vi "Begin.vi"(8 "error in":errorcluster) -> (0 "error out":errorcluster)   [LabVIEW 2014]
doc: "Called before other user functions, this VI is expected to open initial I/O refnums, load in file data, and do all program initialization. Notice that the <B>error out</B> terminal is simply used for data flow. Wiring it to other structures or subVIs ensures that this VI runs first."
uses:
  <vilib>/Rock Robotics/SystemInterfaces/AI/FPGA_AIChannel.ctl
  <vilib>/Rock Robotics/WPI/Solenoid/WPI_SolenoidChannel.ctl
  navX-MXP Library/SERIAL/IO/NI WPI/WPI_SerialPort_USB.ctl
  <vilib>/Rock Robotics/WPI/SafetyOutput/WPI_SafetyOutputConfigMenu.ctl
  <vilib>/Rock Robotics/WPI/Joystick/WPI_JoystickDeviceEnum.ctl
  <vilib>/Rock Robotics/WPI/Compressor/WPI_CompressorGetSetRefNum.vi
  <vilib>/Rock Robotics/WPI/RobotDrive/WPI_RobotDriveOpen4MotorWithCANTalonSRX.vi
  <vilib>/Rock Robotics/WPI/MotorControl/WPI_MotorControlOpenCANTalonSRX.vi
  <vilib>/Rock Robotics/WPI/Solenoid/WPI_SolenoidOpenSingle.vi
  Robot Global Data.vi
  navX-MXP Library/navX-MXP IMU.lvlib
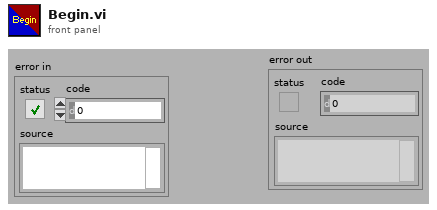
[diagram p1: front panel]
types:
  T1 = typedef "WPI_SolenoidChannel.ctl" = enum8{"Solenoid 0", "Solenoid 1", "Solenoid 2", "Solenoid 3", "Solenoid 4", "Solenoid 5", "Solenoid 6", "Solenoid 7", "Invalid"}
  T2 = typedef "WPI_SolenoidDevRef.ctl" = cluster{"DevStatus":errorcluster, "Pneumatics Control Module":u8, "Forward Solenoid Channel":T1, "Reverse Solenoid Channel":T1}
  T3 = cluster{"String Potentiometer":dbl, "Setpoint":dbl, "Level":sgl}
  T4 = typedef "WPI_CompressorDevRef.ctl" = cluster{"DevStatus":errorcluster, "Pneumatics Control Module":u8}
  T5 = typedef "navX-MXP IMU.lvlib/WPI_SerialPort_USB.ctl" = enum16{"Onboard RS-232", "MXP TTL", "USB"}
  T6 = typedef "navX-MXP IMU.lvlib/navX SPI DevRef.ctl" = cluster{"SPIDevRef":T7, "Board Information":T10, "Status":T11, "Offsets":cluster{"Yaw":dbl, "Quat W":dbl, "Quat X":dbl, "Quat Y":dbl, "Quat Z":dbl}, "Update Rate (4Hz-60Hz)":u8, "refnum name":string, "error":errorcluster}
  T7 = typedef "WPI_SPIDevRef.ctl" = cluster{"DevStatus":errorcluster, "Handle":i32, "Controller":T8, "SPI Bus":T9}
  T8 = typedef "FPGA_TypedefDigitalModule.ctl" = enum16{"Controller 1"}
  T9 = typedef "spi_bus.ctl" = enum16{"SPI On-Board, CS0", "SPI On-Board, CS1", "SPI On-Board, CS2", "SPI On-Board, CS3", "SPI MXP", "Invalid"}
  T10 = typedef "navX-MXP IMU.lvlib/navX Board Information.ctl" = cluster{"WhoAmI (50 | 0x32)":u8, "Board Revision":u8, "Firmware Major Version":u8, "Firmware Minor Version":u8}
  T11 = typedef "navX-MXP IMU.lvlib/navX Status Data.ctl" = cluster{"Update Rate Hz":u8, "Accelerometer Full-Scale Range":u8, "Gyro Full-Scale Range":u16, "NAVX_OP_STATUS":T12, "NAVX_CAL_STATUS":T13, "NAVX_SELFTEST_STATUS":u8, "NAVX_SENSOR_STATUS":T14}
  T12 = typedef "navX-MXP IMU.lvlib/navX NAVX_OP_STATUS.ctl" = u8
  T13 = typedef "navX-MXP IMU.lvlib/navX NAVX_CAL_STATUS.ctl" = u8
  T14 = typedef "navX-MXP IMU.lvlib/navX NAVX_SENSOR_STATUS.ctl" = cluster{"MOVING":bool, "YAW_STABLE":bool, "MAG_DISTURBANCE":bool, "ALTITUDE_VALID":bool, "SEALEVEL_PRESS_SET":bool, "FUSED_HEADING_VALID":bool}
  T15 = typedef "navX-MXP IMU.lvlib/navX Serial DevRef.ctl" = cluster{"SerialPortRef":T16, "Board Information":T10, "Status":T11, "Offsets":cluster{"Yaw":dbl, "Quat W":dbl, "Quat X":dbl, "Quat Y":dbl, "Quat Z":dbl}, "Update Rate (4Hz-60Hz)":u8, "Nav6Mode (YPR)":T17, "refnum name":string, "error":errorcluster}
  T16 = typedef "WPI_SerialPortRef.ctl" = cluster{"DevStatus":errorcluster, "Serial Port Name":refnum<visa-resource-name>}
  T17 = typedef "navX-MXP IMU.lvlib/navX Serial Mode.ctl" = enum16{"YPR", "Gyro", "Quaternion"}
  T18 = typedef "FPGA_AIChannel.ctl" = enum8{"AI 0", "AI 1", "AI 2", "AI 3", "AI MXP 0", "AI MXP 1", "AI MXP 2", "AI MXP 3", "Invalid"}
  T19 = typedef "WPI_AnalogChannelDevRef.ctl" = cluster{"DevStatus":errorcluster, "Controller":T20, "Analog Channel":T18}
  T20 = typedef "FPGA_TypedefAnalogModule.ctl" = enum16{"Controller 1"}
  T21 = typedef "WPI_SafetyOutputConfigMenu.ctl" = enum16{"Enable", "Disable"}
  T22 = typedef "WPI_RobotDriveDevRef.ctl" = cluster{"DevStatus":errorcluster, "Motors[]":T23[], "Square Inputs":bool, "Max Output":dbl}
  T23 = typedef "WPI_MotorControlDeviceRef.ctl" = cluster{"DeviceStatus":errorcluster, "Type":T24, "PWM":cluster{"Controller":T8, "PWM Channel":T25, "DeadBand":T26}, "CAN":cluster{"Device Number":u8, "Control Mode":T27, "Semaphore":T28, "Max Vout":dbl, "TalonSRX Control Mode":T29}, "Invert":bool, "TransformRef":T30, "InvTransformRef":T30}
  T24 = typedef "WPI_MotorControlType.ctl" = enum16{"PWM", "CAN", "CANTalonSRX"}
  T25 = typedef "FPGA_DIOPWMChannel.ctl" = enum8{"PWM 0", "PWM 1", "PWM 2", "PWM 3", "PWM 4", "PWM 5", "PWM 6", "PWM 7", "PWM 8", "PWM 9", "PWM MXP 0", "PWM MXP 1", "PWM MXP 2", "PWM MXP 3", "PWM MXP 4", "PWM MXP 5", "PWM MXP 6", "PWM MXP 7", "PWM MXP 8", "PWM MXP 9", "Invalid"}
  T26 = typedef "WPI_PWMDeadband.ctl" = cluster{"Name":string, "maxPositivePwm":i32, "minPositivePwm":i32, "centerPwm":i32, "maxNegativePwm":i32, "minNegativePwm":i32, "angularRange":u16}
  T27 = typedef "WPI_CANJaguar_ControlMode.ctl" = enum8{"Percent VBus", "Current", "Speed", "Position", "Voltage"}
  T28 = typedef "Semaphore RefNum" = refnum<k1>
  T29 = typedef "WPI_CANTalonSRX_APIControlMode.ctl" = enum8{"Percent VBus", "Speed", "Position", "Slave", "Unchanged / Invalid"}
  T30 = typedef "WPI_PWMTransform_ConPane.ctl" = refnum<vi>
  T31 = typedef "WPI_JoystickDeviceEnum.ctl" = enum16{"USB 0", "USB 1", "USB 2", "USB 3", "USB 4", "USB 5"}
  T32 = typedef "WPI_JoystickDevRef.ctl" = cluster{"Device":T31}
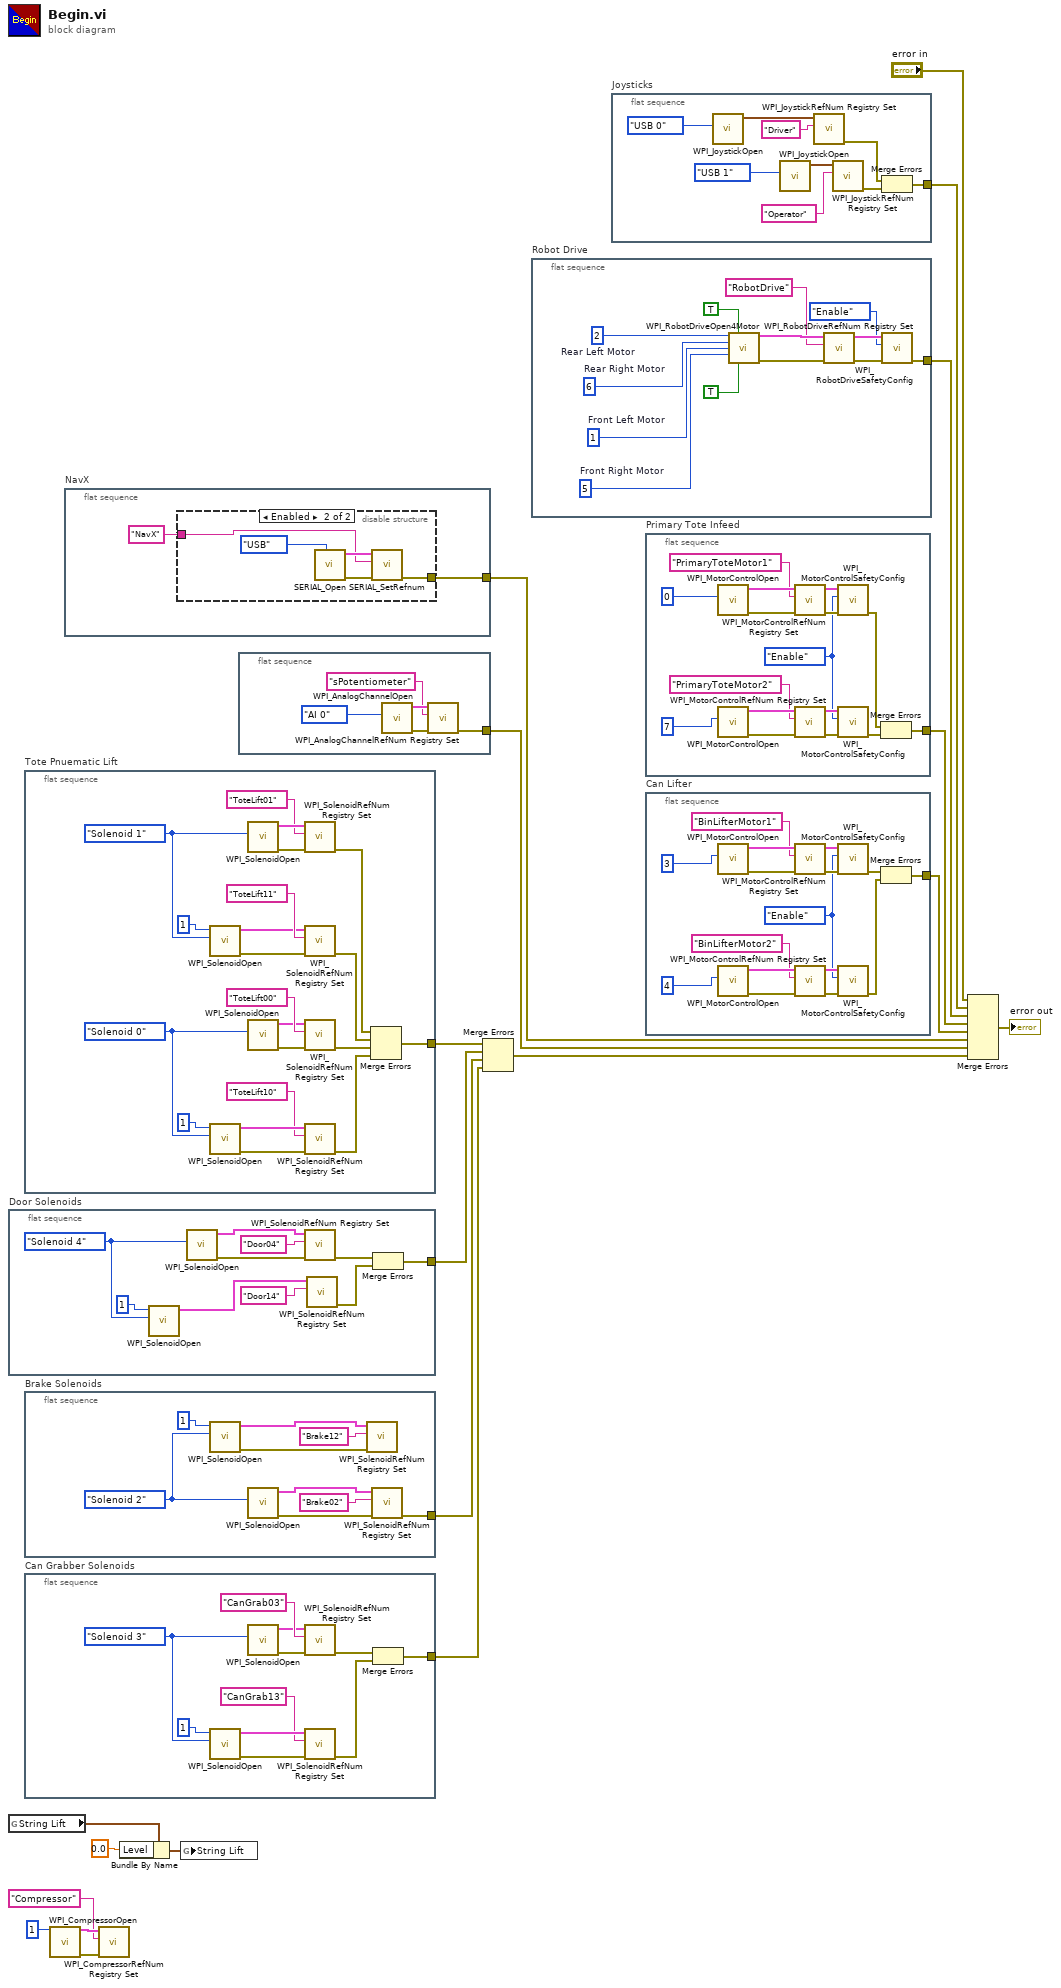
[diagram p0: block diagram]
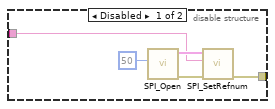
[diagram p2: hidden frame]
diagram:
  n1 = flat-sequence "Door Solenoids" {
    tunnel: [w21] -> w6
    frame #0 {
      w27 = WPI_SolenoidChannel."Solenoid 4" ("Reverse Solenoid Channel")
      n2 = call-poly <vilib>:"WPI_SolenoidOpen.vi"("Solenoid Channel"=w27, "Pneumatics Control Module (0)"=u8 1) -> ("SolenoidDevRef"=w26:T2)  [unwired: 8 in, 1 out]
      n3 = call-poly <vilib>:"WPI_SolenoidOpen.vi"("Solenoid Channel"=w27) -> ("error out"=w24:errorcluster, "SolenoidDevRef"=w25:T2)  [unwired: 9 in]
      n4 = call <vilib>:"WPI_SolenoidRefNum Registry Set.vi"("error in (no error)"=w24, "refnum name"="Door04", "SolenoidDevRef"=w25) -> ("error out"=w23:errorcluster)  [unwired: 7 in, 1 out]
      n5 = call <vilib>:"WPI_SolenoidRefNum Registry Set.vi"("refnum name"="Door14", "SolenoidDevRef"=w26) -> ("error out"=w22:errorcluster)  [unwired: 8 in, 1 out]
      n6 = Merge Errors(w23, w22) -> (w21:errorcluster)
    }
  }
  n7 = global read "Robot Global Data.vi" "String Lift"() -> (w3:T3)
  n8 = flat-sequence "Tote Pnuematic Lift" {
    tunnel: [w34] -> w5
    frame #0 {
      w38 = WPI_SolenoidChannel."Solenoid 1" ("Forward Solenoid Channel")
      w45 = WPI_SolenoidChannel."Solenoid 0" ("Forward Solenoid Channel")
      n9 = call-poly <vilib>:"WPI_SolenoidOpen.vi"("Solenoid Channel"=w38, "Pneumatics Control Module (0)"=u8 1) -> ("error out"=w39:errorcluster, "SolenoidDevRef"=w40:T2)  [unwired: 8 in]
      n10 = call-poly <vilib>:"WPI_SolenoidOpen.vi"("Solenoid Channel"=w45, "Pneumatics Control Module (0)"=u8 1) -> ("error out"=w51:errorcluster, "SolenoidDevRef"=w50:T2)  [unwired: 8 in]
      n11 = call-poly <vilib>:"WPI_SolenoidOpen.vi"("Solenoid Channel"=w38) -> ("error out"=w44:errorcluster, "SolenoidDevRef"=w43:T2)  [unwired: 9 in]
      n12 = call-poly <vilib>:"WPI_SolenoidOpen.vi"("Solenoid Channel"=w45) -> ("error out"=w46:errorcluster, "SolenoidDevRef"=w47:T2)  [unwired: 9 in]
      n13 = call <vilib>:"WPI_SolenoidRefNum Registry Set.vi"("error in (no error)"=w44, "refnum name"="ToteLift01", "SolenoidDevRef"=w43) -> ("error out"=w33:errorcluster)  [unwired: 7 in, 1 out]
      n14 = call <vilib>:"WPI_SolenoidRefNum Registry Set.vi"("error in (no error)"=w39, "refnum name"="ToteLift11", "SolenoidDevRef"=w40) -> ("error out"=w32:errorcluster)  [unwired: 7 in, 1 out]
      n15 = call <vilib>:"WPI_SolenoidRefNum Registry Set.vi"("error in (no error)"=w46, "refnum name"="ToteLift00", "SolenoidDevRef"=w47) -> ("error out"=w31:errorcluster)  [unwired: 7 in, 1 out]
      n16 = call <vilib>:"WPI_SolenoidRefNum Registry Set.vi"("error in (no error)"=w51, "refnum name"="ToteLift10", "SolenoidDevRef"=w50) -> ("error out"=w35:errorcluster)  [unwired: 7 in, 1 out]
      n17 = Merge Errors(w33, w32, w31, w35) -> (w34:errorcluster)
    }
  }
  n18 = flat-sequence "Brake Solenoids" {
    tunnel: [w57] -> w7
    frame #0 {
      w53 = WPI_SolenoidChannel."Solenoid 2" ("Reverse Solenoid Channel")
      n19 = call-poly <vilib>:"WPI_SolenoidOpen.vi"("Solenoid Channel"=w53, "Pneumatics Control Module (0)"=u8 1) -> ("error out"=w56:errorcluster, "SolenoidDevRef"=w52:T2)  [unwired: 8 in]
      n20 = call-poly <vilib>:"WPI_SolenoidOpen.vi"("Solenoid Channel"=w53) -> ("error out"=w58:errorcluster, "SolenoidDevRef"=w59:T2)  [unwired: 9 in]
      n21 = call <vilib>:"WPI_SolenoidRefNum Registry Set.vi"("error in (no error)"=w56, "refnum name"="Brake12", "SolenoidDevRef"=w52) -> ()  [unwired: 7 in, 2 out]
      n22 = call <vilib>:"WPI_SolenoidRefNum Registry Set.vi"("error in (no error)"=w58, "refnum name"="Brake02", "SolenoidDevRef"=w59) -> ("error out"=w57:errorcluster)  [unwired: 7 in, 1 out]
    }
  }
  n23 = flat-sequence "Can Grabber Solenoids" {
    tunnel: [w61] -> w8
    frame #0 {
      w70 = WPI_SolenoidChannel."Solenoid 3" ("Reverse Solenoid Channel")
      n24 = call-poly <vilib>:"WPI_SolenoidOpen.vi"("Solenoid Channel"=w70, "Pneumatics Control Module (0)"=u8 1) -> ("error out"=w69:errorcluster, "SolenoidDevRef"=w68:T2)  [unwired: 8 in]
      n25 = call-poly <vilib>:"WPI_SolenoidOpen.vi"("Solenoid Channel"=w70) -> ("error out"=w64:errorcluster, "SolenoidDevRef"=w65:T2)  [unwired: 9 in]
      n26 = call <vilib>:"WPI_SolenoidRefNum Registry Set.vi"("error in (no error)"=w64, "refnum name"="CanGrab03", "SolenoidDevRef"=w65) -> ("error out"=w63:errorcluster)  [unwired: 7 in, 1 out]
      n27 = call <vilib>:"WPI_SolenoidRefNum Registry Set.vi"("error in (no error)"=w69, "refnum name"="CanGrab13", "SolenoidDevRef"=w68) -> ("error out"=w62:errorcluster)  [unwired: 7 in, 1 out]
      n28 = Merge Errors(w63, w62) -> (w61:errorcluster)
    }
  }
  n29 = call <vilib>:"WPI_CompressorOpen.vi"("Pneumatics Control Module (0)"=u8 1) -> ("CompressorDevRef"=w11:T4, "error out"=w12:errorcluster)  [unwired: 13 in]
  n30 = flat-sequence "NavX" {
    tunnel: [w73] -> w14
    frame #0 {
      n31 = disable-structure shown="Enabled" {
        disable-tunnel: [w75 w79] -> w73
        disable-tunnel: "NavX" ("refnum name") -> [w74 w80]
        frame Disabled {
          n32 = call "SPI_Open.vi"("Update Rate (4Hz-60Hz)"=u8 50) -> ("error out"=w77:errorcluster, "navX DevRef"=w76:T6)  [unwired: 8 in, 1 out]
          n33 = call "SPI_SetRefnum.vi"("error in (no error)"=w77, "refnum name"=w74, "navX DevRef"=w76) -> ("error out"=w75:errorcluster)  [unwired: 7 in, 1 out]
        }
        frame Enabled {
          n34 = call "SERIAL_Open.vi"("Serial Port (MXP)"=WPI_SerialPort_USB."USB") -> ("error out"=w83:errorcluster, "navX Ref"=w82:T15)  [unwired: 8 in, 1 out]
          n35 = call "SERIAL_SetRefnum.vi"("error in (no error)"=w83, "refnum name"=w80, "navX DevRef"=w82) -> ("error out"=w79:errorcluster)  [unwired: 7 in, 1 out]
        }
      }
    }
  }
  n36 = call <vilib>:"WPI_CompressorRefNum Registry Set.vi"("error in (no error)"=w12, "refnum name"="Compressor", "CompressorDevRef"=w11) -> ()  [unwired: 7 in, 2 out]
  n37 = Bundle By Name(cluster=w3, "Level"=sgl 0.0) -> (w2:T3)
  n38 = global write "Robot Global Data.vi" "String Lift"(w2) -> ()
  n39 = flat-sequence {
    tunnel: [w86] -> w9
    frame #0 {
      n40 = call <vilib>:"WPI_AnalogChannelOpen.vi"("Analog Channel"=FPGA_AIChannel."AI 0") -> ("error out"=w87:errorcluster, "AIDeviceRef"=w88:T19)  [unwired: 9 in]
      n41 = call <vilib>:"WPI_AnalogChannelRefNum Registry Set.vi"("error in (no error)"=w87, "refnum name"="sPotentiometer", "AIDeviceRef"=w88) -> ("error out"=w86:errorcluster)  [unwired: 7 in, 1 out]
    }
  }
  n42 = Merge Errors(w5, w6, w7, w8) -> (w4:errorcluster)
  n43 = flat-sequence "Robot Drive" {
    tunnel: [w91] -> w20
    frame #0 {
      w98 = u8 5  # Front Right Motor
      w99 = u8 1  # Front Left Motor
      w100 = u8 6  # Rear Right Motor
      w101 = u8 2  # Rear Left Motor
      n44 = call-poly <vilib>:"WPI_RobotDriveOpen4Motor.vi"("Rear Left Motor"=w101, "Rear Left Motor Inverted"=TRUE, "Rear Right Motor"=w100, "Front Left Motor"=w99, "Front Right Motor"=w98, "Front Left Motor Inverted"=TRUE) -> ("RobotDriveDevRef"=w97:T22, "error out"=w96:errorcluster)  [unwired: 8 in]
      n45 = call <vilib>:"WPI_RobotDriveRefNum Registry Set.vi"("error in (no error)"=w96, "refnum name"="RobotDrive", "RobotDriveDevRef"=w97) -> ("error out"=w93:errorcluster, "RobotDriveDevRef"=w94:T22)  [unwired: 7 in]
      n46 = call <vilib>:"WPI_RobotDriveSafetyConfig.vi"("error in (no error)"=w93, "mode"=WPI_SafetyOutputConfigMenu."Enable", "RobotDriveDevRef"=w94) -> ("error out"=w91:errorcluster)  [unwired: 7 in, 1 out]
    }
  }
  n47 = flat-sequence "Joysticks" {
    tunnel: [w106] -> w19
    frame #0 {
      n48 = call <vilib>:"WPI_JoystickOpen.vi"("JoystickDevice"=WPI_JoystickDeviceEnum."USB 0") -> ("JoystickDevRef"=w108:T32)  [unwired: 10 in]
      n49 = call <vilib>:"WPI_JoystickOpen.vi"("JoystickDevice"=WPI_JoystickDeviceEnum."USB 1") -> ("JoystickDevRef"=w104:T32)  [unwired: 10 in]
      n50 = call <vilib>:"WPI_JoystickRefNum Registry Set.vi"("refnum name"="Driver", "JoystickDevRef"=w108) -> ("error out"=w107:errorcluster)  [unwired: 8 in, 1 out]
      n51 = call <vilib>:"WPI_JoystickRefNum Registry Set.vi"("refnum name"="Operator", "JoystickDevRef"=w104) -> ("error out"=w102:errorcluster)  [unwired: 8 in, 1 out]
      n52 = Merge Errors(w107, w102) -> (w106:errorcluster)
    }
  }
  n53 = flat-sequence "Primary Tote Infeed" {
    tunnel: [w115] -> w18
    frame #0 {
      w112 = WPI_SafetyOutputConfigMenu."Enable" ("mode")
      n54 = call-poly <vilib>:"WPI_MotorControlOpen.vi"("Device Number"=u8 0) -> ("error out"=w125:errorcluster, "MotorControlDeviceRef"=w124:T23)  [unwired: 9 in]
      n55 = call-poly <vilib>:"WPI_MotorControlOpen.vi"("Device Number"=u8 7 ("Master Device Number")) -> ("error out"=w123:errorcluster, "MotorControlDeviceRef"=w122:T23)  [unwired: 9 in]
      n56 = call <vilib>:"WPI_MotorControlRefNum Registry Set.vi"("error in (no error)"=w125, "refnum name"="PrimaryToteMotor1", "MotorControlDevRef"=w124) -> ("error out"=w120:errorcluster, "MotorControlDevRef"=w121:T23)  [unwired: 7 in]
      n57 = call <vilib>:"WPI_MotorControlRefNum Registry Set.vi"("error in (no error)"=w123, "refnum name"="PrimaryToteMotor2", "MotorControlDevRef"=w122) -> ("error out"=w119:errorcluster, "MotorControlDevRef"=w118:T23)  [unwired: 7 in]
      n58 = call <vilib>:"WPI_MotorControlSafetyConfig.vi"("error in (no error)"=w120, "mode"=w112, "MotorControlDevRef"=w121) -> ("error out"=w117:errorcluster)  [unwired: 7 in, 1 out]
      n59 = call <vilib>:"WPI_MotorControlSafetyConfig.vi"("error in (no error)"=w119, "mode"=w112, "MotorControlDevRef"=w118) -> ("error out"=w116:errorcluster)  [unwired: 7 in, 1 out]
      n60 = Merge Errors(w117, w116) -> (w115:errorcluster)
    }
  }
  n61 = flat-sequence "Can Lifter" {
    tunnel: [w132] -> w17
    frame #0 {
      w129 = WPI_SafetyOutputConfigMenu."Enable" ("mode")
      n62 = call-poly <vilib>:"WPI_MotorControlOpen.vi"("Device Number"=u8 3 ("Master Device Number")) -> ("error out"=w142:errorcluster, "MotorControlDeviceRef"=w141:T23)  [unwired: 9 in]
      n63 = call-poly <vilib>:"WPI_MotorControlOpen.vi"("Device Number"=u8 4 ("Master Device Number")) -> ("error out"=w140:errorcluster, "MotorControlDeviceRef"=w139:T23)  [unwired: 9 in]
      n64 = call <vilib>:"WPI_MotorControlRefNum Registry Set.vi"("error in (no error)"=w142, "refnum name"="BinLifterMotor1", "MotorControlDevRef"=w141) -> ("error out"=w138:errorcluster, "MotorControlDevRef"=w137:T23)  [unwired: 7 in]
      n65 = call <vilib>:"WPI_MotorControlRefNum Registry Set.vi"("error in (no error)"=w140, "refnum name"="BinLifterMotor2", "MotorControlDevRef"=w139) -> ("error out"=w136:errorcluster, "MotorControlDevRef"=w135:T23)  [unwired: 7 in]
      n66 = call <vilib>:"WPI_MotorControlSafetyConfig.vi"("error in (no error)"=w138, "mode"=w129, "MotorControlDevRef"=w137) -> ("error out"=w134:errorcluster)  [unwired: 7 in, 1 out]
      n67 = call <vilib>:"WPI_MotorControlSafetyConfig.vi"("error in (no error)"=w136, "mode"=w129, "MotorControlDevRef"=w135) -> ("error out"=w133:errorcluster)  [unwired: 7 in, 1 out]
      n68 = Merge Errors(w134, w133) -> (w132:errorcluster)
    }
  }
  n69 = Merge Errors("error in", w19, w20, w18, w17, w14, w9, w4) -> (→"error out":errorcluster)
